vi "Set Interface Settings.vi"(10 "Interface Settings":T1, 11 "Model in":refnum<class "Model.lvclass">) -> (3 "Model out":refnum<class "Model.lvclass">)   [LabVIEW 2016, in "Model.lvclass"]
uses:
  Model.lvclass
  Typedefs/TestSettings.ctl
  Model.lvclass/Model.ctl
  Typedefs/M1M3SupportEUI_TypeDefs.lvlib
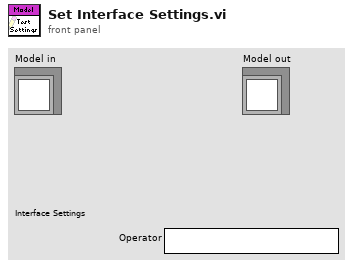
[diagram p1: front panel]
types:
  T1 = typedef "M1M3SupportEUI_TypeDefs.lvlib/TestSettings.ctl" = cluster{"Operator":string}
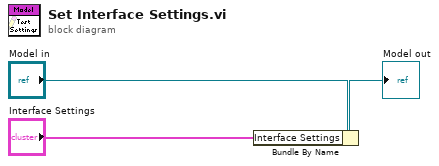
[diagram p0: block diagram]
diagram:
  n1 = Bundle By Name(cluster="Model in", "Interface Settings"="Interface Settings") -> (→"Model out":refnum<class "Model.lvclass">)
